vi "Close NISE Session.vi"(8 "error in (no error)":errorcluster, 11 "UI Data in":T1) -> (0 "error out":errorcluster, 3 "UI Data out":T1)   [LabVIEW 2025, in "Switch Executive Controller UI.lvlib"]
uses:
  Switch Executive Controller UI.lvlib
  <vilib>/SwitchExecutive/nise.llb/niSE SessionRefnum.ctl
  UI Data.ctl
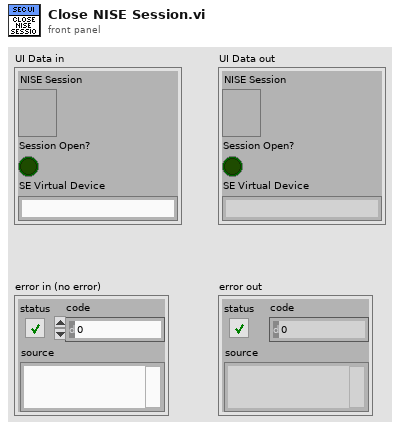
[diagram p1: front panel]
types:
  T1 = typedef "Switch Executive Controller UI.lvlib/UI Data.ctl" = cluster{"NISE Session":T2, "Session Open?":bool, "SE Virtual Device":string}
  T2 = typedef "niSE SessionRefnum.ctl" = refnum<k1>
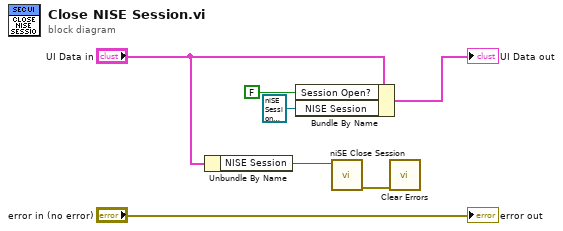
[diagram p0: block diagram]
diagram:
  n1 = Unbundle By Name("UI Data in") -> ("NISE Session"=w3:T2)
  n2 = Bundle By Name(cluster="UI Data in", "Session Open?"=FALSE, "NISE Session"=T2 refnum) -> (→"UI Data out":T1)
  n3 = call <vilib>:"niSE Close Session.vi"("NISE Session (in)"=w3) -> ("error out"=w4:errorcluster)  [unwired: 6 in]
  n4 = call <vilib>:"Clear Errors.vi"("error in (no error)"=w4) -> ()  [unwired: 5 in, 2 out]
  "error out" <- "error in (no error)"
